vi "stream name to fifo names.vi"(11 "Name":string) -> (1 "data to CD":string, 2 "meta to CD":string, 3 "meta from CD":string)   [LabVIEW 2026, in "Nominal Core Streaming Shared.lvlib"]
uses:
  Nominal Core Streaming Shared.lvlib
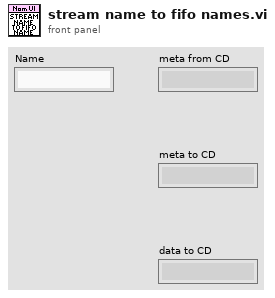
[diagram p1: front panel]
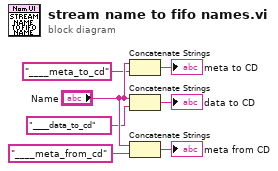
[diagram p0: block diagram]
diagram:
  n1 = Concatenate Strings("Name", "____meta_to_cd" ("string")) -> (→"meta to CD":string)
  n2 = Concatenate Strings("Name", "____data_to_cd" ("string")) -> (→"data to CD":string)
  n3 = Concatenate Strings("Name", "____meta_from_cd" ("string")) -> (→"meta from CD":string)
